vi "Error 7002.vi"(8 "error in (no error)":errorcluster, 10 "VI name in":string, 11 "Packekd library name in":string) -> (0 "error out":errorcluster)   [LabVIEW 2019, in "LVLIBP CD XML Updater.lvlib"]
uses:
  LVLIBP CD XML Updater.lvlib
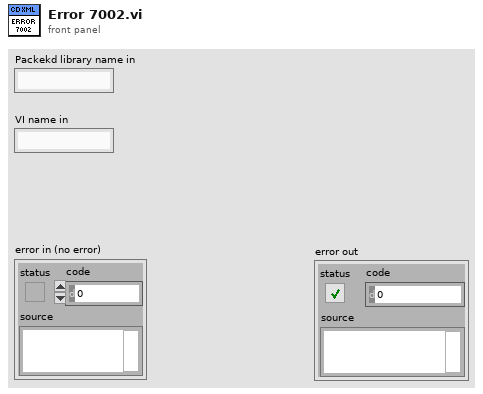
[diagram p1: front panel]
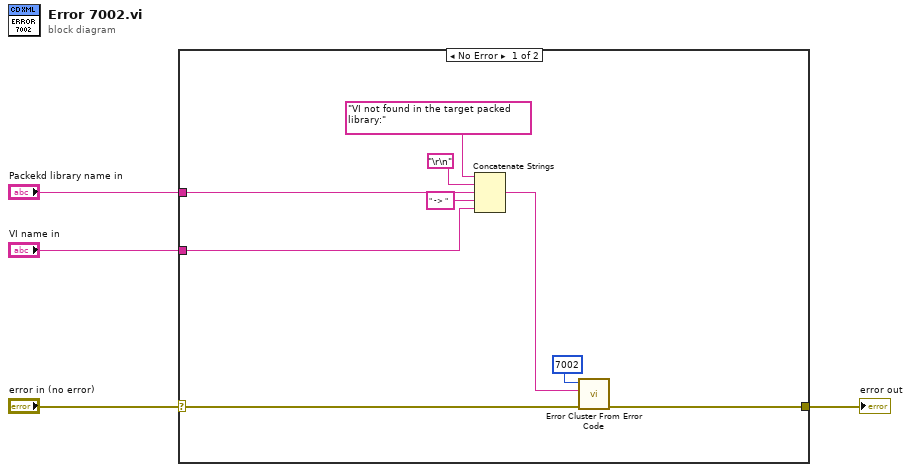
[diagram p0: block diagram]
diagram:
  n1 = case shown="No Error" "error in (no error)" {
    selector: "error in (no error)" -> [w13 w14]
    tunnel: [w12 w14] -> w3
    tunnel: "VI name in" -> [w5 _]
    tunnel: "Packekd library name in" -> [w7 _]
    frame No Error {
      n2 = Concatenate Strings("VI not found in the target packed library:" ("error message (\"\")"), "\r\n", w7, " -> " ("string"), w5) -> (w9:string)
      n3 = call <vilib>:"Error Cluster From Error Code.vi"("error in (no error)"=w13, "error message (\"\")"=w9, "error code (0)"=7002) -> ("error out"=w12:errorcluster)  [unwired: 6 in]
    }
    frame Error {
    }
  }
  "error out" <- w3
